vi "PrefDialog.vi"(8 "error in (no error)":errorcluster, 11 "DigitizerBase":refnum<class "DigitizerBase.lvclass">) -> (0 "error out":errorcluster, 3 "DigitizerBase":refnum<class "DigitizerBase.lvclass">)   [LabVIEW 2018, in "DigitizerPlugins.lvlib" / "DigitizerBase.lvclass"]
uses:
  DigitizerBase.lvclass
  C:/Program Files/National Instruments/LabVIEW 2018/user.lib/NIST/BaseClasses/BasePlugin_class/BasePlugin.lvclass
  Typedefs/Acquisition.ctl
  Typedefs/Channel.ctl
  Typedefs/Trigger.ctl
  Typedefs/TrigSource.ctl
  DigitizerBase.lvclass/DigitizerBase.ctl
  <userlib>/NIST/BaseClasses/BasePlugin_class/BasePlugin.lvclass/BasePlugin.ctl
  Accessors/Read Acquisition.vi
  Accessors/Read Channels.vi
  Accessors/Read Trigger.vi
  <userlib>/NIST/BaseClasses/BasePlugin_class/Accessors/Read PluginIniFilePath.vi
  Accessors/Write Acquisition.vi
  Accessors/Write Trigger.vi
  Accessors/Write Channels.vi
  <userlib>/NIST/BaseClasses/BasePlugin_class/Accessors/Write PluginIniFilePath.vi
  <vilib>/Utility/config.llb/NI_LVConfig.lvlib
panel:
  in  "btnSaveAs":bool
  in  "Trigger":T1
  in  "Channels":T3[](array[typedef])
  in  "Acquisition":T4 {"SampleMode" items=["Real Time", "Equivalent Time"]}
  in  "btnSave":bool
  in  "btnCancel":bool
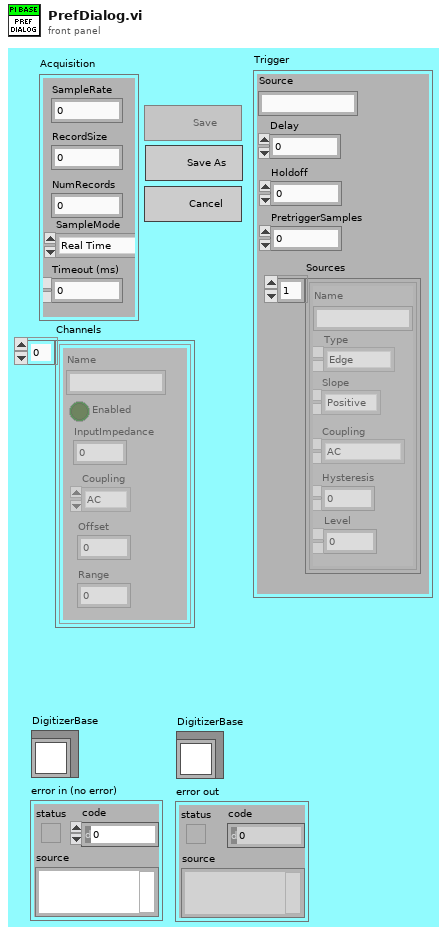
[diagram p1: front panel]
types:
  T1 = typedef "DigitizerPlugins.lvlib/DigitizerBase.lvclass/Trigger.ctl" = cluster{"Source":string, "Delay":dbl, "Holdoff":dbl, "PretriggerSamples":i32, "Sources":T2[]}
  T2 = typedef "DigitizerPlugins.lvlib/DigitizerBase.lvclass/TrigSource.ctl" = cluster{"Name":string, "Coupling":enum16{"AC", "DC", "HF Reject", "LF Reject", "Noise Reject"}, "Hysteresis":dbl, "Level":dbl, "Slope":enum16{"Positive", "Negative"}, "Type":enum16{"Edge", "Width", "Runt", "Glitch", "TV", "Window"}}
  T3 = typedef "DigitizerPlugins.lvlib/DigitizerBase.lvclass/Channel.ctl" = cluster{"Name":string, "Enabled":bool, "InputImpedance":dbl, "Coupling":enum16{"AC", "DC", "Gnd"}, "Offset":dbl, "Range":dbl}
  T4 = typedef "DigitizerPlugins.lvlib/DigitizerBase.lvclass/Acquisition.ctl" = cluster{"SampleRate":dbl, "RecordSize":i32, "NumRecords":i32, "SampleMode":i32, "Timeout (ms)":i32}
  T5 = enum8{"Enabled", "Disabled", "Disabled and Grayed Out"}
  T6 = enum32{"Invalid", "Default", "Floating", "Floating/Auto-Hide", "Modal"}
  T7 = typedef "NI_LVConfig.lvlib/Config Data RefNum.ctl" = refnum<k1>
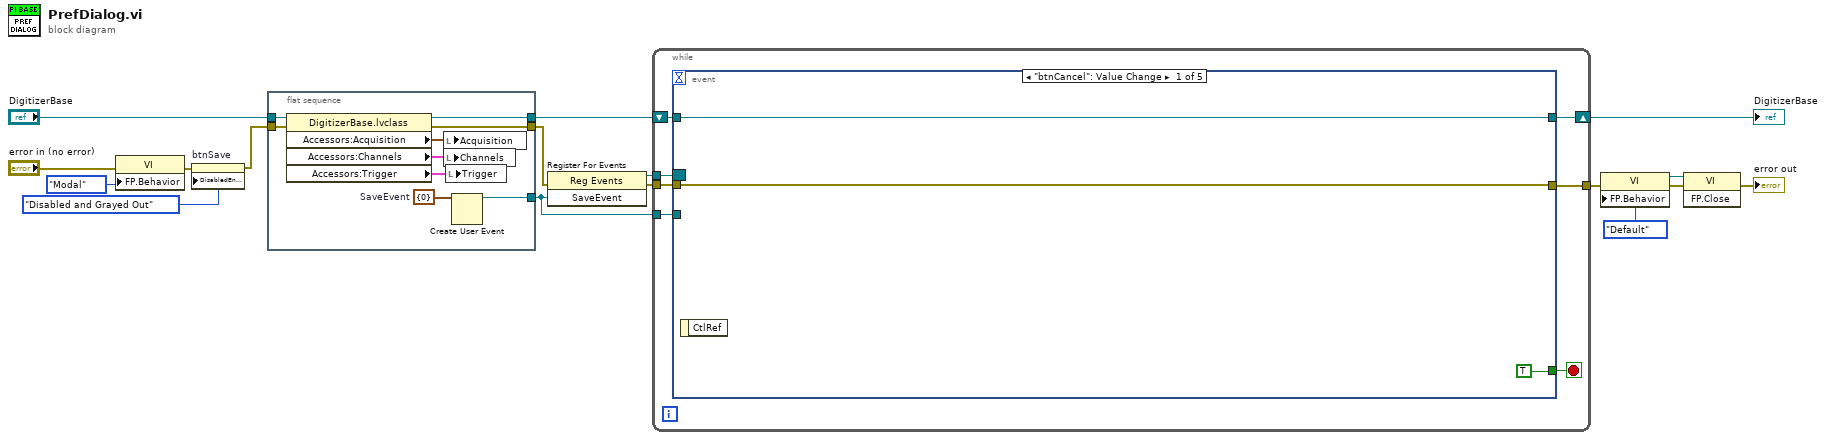
[diagram p0: block diagram]
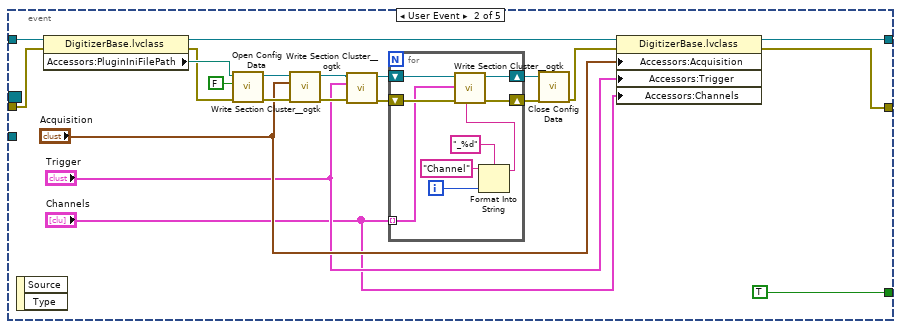
[diagram p2: hidden frame]
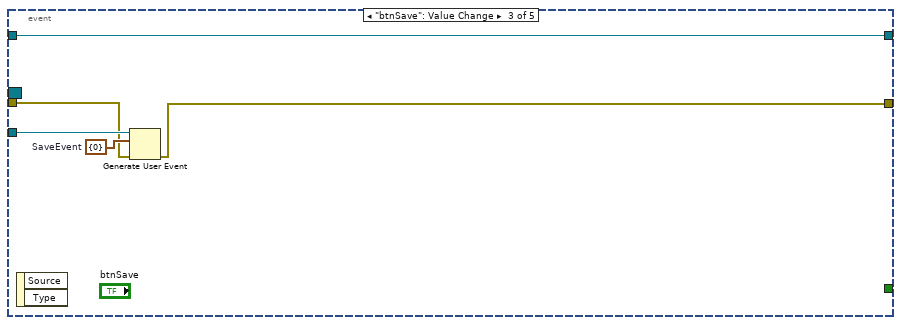
[diagram p3: hidden frame]
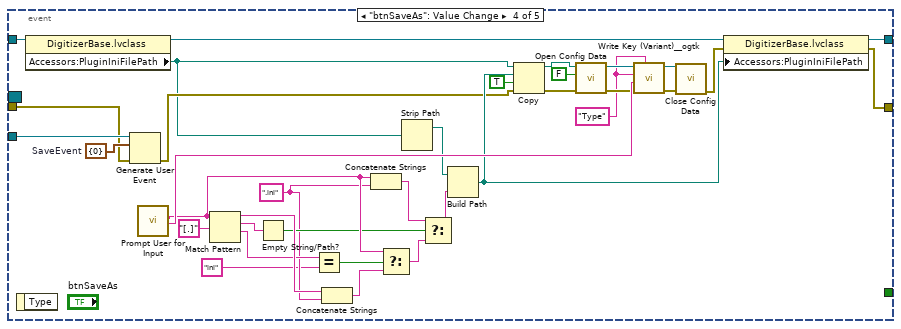
[diagram p4: hidden frame]
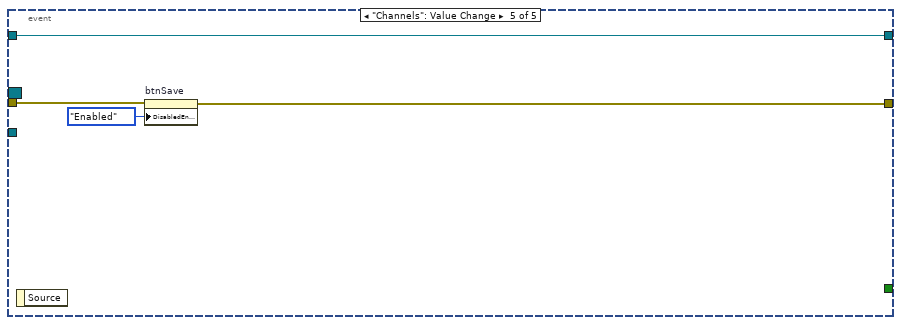
[diagram p5: hidden frame]
diagram:
  n1 = property class="VI"(error in="error in (no error)", "FP.Behavior"=T6."Modal" ("Front Panel Window:Behavior")) -> (error out=w3:errorcluster)  [unwired: 1 in, 1 out]
  n2 = property on="btnSave" class="Bool"(error in=w3, "DisabledEnum"=T5."Disabled and Grayed Out" ("Disabled")) -> (error out=w2:errorcluster)  [unwired: 1 in, 1 out]
  n3 = flat-sequence {
    tunnel: "DigitizerBase" -> [w26]
    tunnel: [w25] -> w9
    tunnel: w2 -> [w22]
    tunnel: [w19] -> w6
    tunnel: [w18] -> w4
    frame #0 {
      w20 = cluster{"Num":i32} {"Num"=0}  # SaveEvent
      n4 = property class="DigitizerBase.lvclass"(reference=w26, error in=w22) -> (reference out=w25:refnum<class "DigitizerBase.lvclass">, error out=w19:errorcluster, "Accessors:Acquisition"=w24:T4, "Accessors:Channels"=w21:T3[], "Accessors:Trigger"=w23:T1)
      n5 = local write "Acquisition"(w24) -> ()
      n6 = local write "Channels"(w21) -> ()
      n7 = local write "Trigger"(w23) -> ()
      n8 = Create User Event(user event datatype=w20) -> (user event=w18:refnum<user-event>)  [unwired: 1 in, 1 out]
    }
  }
  n9 = register-events(error in=w6, w4) -> (reference out=w7:refnum<event-registration>, error out=w5:errorcluster)  [unwired: 1 in]
  n10 = while {
    tunnel: w7 -> [w29]
    shift-right: [w33] -> w17
    shift-left: w9 -> [w31]
    tunnel: w5 -> [w30]
    tunnel: [w32] -> w15
    tunnel: w4 -> [w27]
    stop <- w28 stop-if-true
    n11 = event shown="[0] \"btnCancel\": Value Change" {
      selector: w29 -> [_ _ _ _ _]
      dyn-events: _ -> [_ _ _ _ _]
      timeout: _ -> [_ _ _ _ _]
      tunnel: w31 -> [w36 w57 w68 w103 w107]
      tunnel: [w36 w44 w68 w77 w107] -> w33
      tunnel: [w35 w42 w67 w76 w109] -> w32
      tunnel: w30 -> [w35 w38 w69 w104 w110]
      tunnel: [TRUE TRUE _ _ _] -> w28
      tunnel: w27 -> [_ _ w71 w106 _]
      event "btnCancel": Value Change {
        n12 = event-data() -> ()  [unwired: 1 in, 1 out]
      }
      event User Event {
        n13 = event-data() -> ()  [unwired: 1 in, 2 out]
        n14 = property class="DigitizerBase.lvclass"(reference=w57, error in=w38) -> (reference out=w45:refnum<class "DigitizerBase.lvclass">, error out=w54:errorcluster, "Accessors:PluginIniFilePath"=w56:path)
        n15 = call <vilib>:"Open Config Data.vi"("error in (no error)"=w54, "create file if necessary (T)"=FALSE, "configuration file path"=w56) -> ("error out"=w52:errorcluster, "refnum"=w53:T7)  [unwired: 6 in, 1 out]
        n16 = call <userlib>:"Write Section Cluster__ogtk.vi"("error in (no error)"=w52, "Section Formatted Cluster"="Acquisition", "refnum"=w53) -> ("error out"=w50:errorcluster, "dup refnum"=w51:T7)  [unwired: 7 in]
        n17 = call <userlib>:"Write Section Cluster__ogtk.vi"("error in (no error)"=w50, "Section Formatted Cluster"="Trigger", "refnum"=w51) -> ("error out"=w49:errorcluster, "dup refnum"=w48:T7)  [unwired: 7 in]
        n18 = for {
          shift-right: [w64] -> w47
          shift-left: w49 -> [w66]
          shift-right: [w63] -> w46
          shift-left: w48 -> [w65]
          tunnel: "Channels" -> [w59] mode=indexing
          i -> [w60]
          n19 = Format Into String(format string="_%d", initial string="Channel", w60) -> (resulting string=w58:string)  [unwired: 1 in, 1 out]
          n20 = call <userlib>:"Write Section Cluster__ogtk.vi"("section (optional)"=w58, "error in (no error)"=w66, "Section Formatted Cluster"=w59, "refnum"=w65) -> ("error out"=w64:errorcluster, "dup refnum"=w63:T7)  [unwired: 6 in]
        }
        n21 = call <vilib>:"Close Config Data.vi"("error in (no error)"=w47, "refnum"=w46) -> ("error out"=w43:errorcluster)  [unwired: 8 in, 1 out]
        n22 = property class="DigitizerBase.lvclass"(reference=w45, error in=w43, "Accessors:Acquisition"="Acquisition", "Accessors:Trigger"="Trigger", "Accessors:Channels"="Channels") -> (reference out=w44:refnum<class "DigitizerBase.lvclass">, error out=w42:errorcluster)
      }
      event "btnSave": Value Change {
        w70 = cluster{"Num":i32} {"Num"=0}  # SaveEvent
        n23 = event-data() -> ()  [unwired: 1 in, 2 out]
        n24 = Generate User Event(user event=w71, event data cluster=w70, error in=w69) -> (error out=w67:errorcluster)  [unwired: 1 in, 1 out]
      }
      event "btnSaveAs": Value Change {
        w83 = "Type" ("key (optional)")
        w81 = ".ini" ("string")
        w105 = cluster{"Num":i32} {"Num"=0}  # SaveEvent
        n25 = event-data() -> ()  [unwired: 1 in, 1 out]
        n26 = property class="DigitizerBase.lvclass"(reference=w103) -> (reference out=w78:refnum<class "DigitizerBase.lvclass">, "Accessors:PluginIniFilePath"=w72:path)  [unwired: 1 in, 1 out]
        n27 = Generate User Event(user event=w106, event data cluster=w105, error in=w104) -> (error out=w73:errorcluster)  [unwired: 1 in, 1 out]
        n28 = call "Prompt User for Input"() -> ("File Name"=w94:string, "PluginType Name"=w99:string)  [unwired: 16 in, 2 out]
        n29 = Match Pattern(string=w94, regular expression="[.]" ("string")) -> (before substring=w92:string, match substring=w90:string, after substring=w91:string)  [unwired: 1 in, 1 out]
        n30 = Empty String/Path?(string/path=w90) -> (empty?=w86:bool)
        n31 = Equal?(x=w91, y="ini" ("string")) -> (x = y?=w88:bool)
        n32 = Concatenate Strings(w92, w81) -> (w93:string)
        n33 = Concatenate Strings(w94, w81) -> (w87:string)
        n34 = Select(t=w94, s=w88, f=w93) -> (s? t:f=w89:string)
        n35 = Strip Path(path=w72) -> (stripped path=w95:path)  [unwired: 1 out]
        n36 = Select(t=w87, s=w86, f=w89) -> (s? t:f=w85:string)
        n37 = Build Path(base path=w95, name or relative path=w85) -> (appended path=w74:path)
        n38 = Copy(8:w73, 9:TRUE ("overwrite (F)"), 10:w74, 11:w72) -> (0:w98:errorcluster, 3:w100:path)  [unwired: 1 in, 1 out]
        n39 = call <vilib>:"Open Config Data.vi"("error in (no error)"=w98, "create file if necessary (T)"=FALSE, "configuration file path"=w100) -> ("error out"=w97:errorcluster, "refnum"=w101:T7)  [unwired: 6 in, 1 out]
        n40 = call <userlib>:"Write Key (Variant)__ogtk.vi"("section"=w83, "error in (no error)"=w97, "key-value"=w99, "key (optional)"=w83, "refnum"=w101) -> ("error out"=w96:errorcluster, "refnum out"=w102:T7)  [unwired: 5 in]
        n41 = call <vilib>:"Close Config Data.vi"("error in (no error)"=w96, "refnum"=w102) -> ("error out"=w75:errorcluster)  [unwired: 8 in, 1 out]
        n42 = property class="DigitizerBase.lvclass"(reference=w78, error in=w75, "Accessors:PluginIniFilePath"=w74) -> (reference out=w77:refnum<class "DigitizerBase.lvclass">, error out=w76:errorcluster)
      }
      event "Channels": Value Change {
        n43 = event-data() -> ()  [unwired: 1 in, 1 out]
        n44 = property on="btnSave" class="Bool"(error in=w110, "DisabledEnum"=T5."Enabled" ("Disabled")) -> (error out=w109:errorcluster)  [unwired: 1 in, 1 out]
      }
    }
  }
  "DigitizerBase" <- w17
  n45 = property class="VI"(error in=w15, "FP.Behavior"=T6."Default" ("Front Panel Window:Behavior")) -> (reference out=w11:refnum<vi>, error out=w14:errorcluster)  [unwired: 1 in]
  n46 = invoke class="VI" method="FP.Close"(reference=w11, error in=w14) -> (error out=→"error out":errorcluster)  [unwired: 1 in, 2 out]
